vi "testToChangeGainByPSSN.vi"(8 "error in (no error)":errorcluster) -> (0 "error out":errorcluster)   [LabVIEW 2016]
doc: "Test to change the gain value based on the normalized point source sensitivity (PSSN)."
uses:
  ZTAAC/ZTAAC.lvclass
  <vilib>/addons/_JKI Toolkits/Caraya/classes/Test/Test.lvclass
  <vilib>/addons/_JKI Toolkits/Caraya/classes/Assert/Assert.lvclass
panel:
  in  "ZTAAC.lvclass":refnum<class "ZTAAC.lvclass">
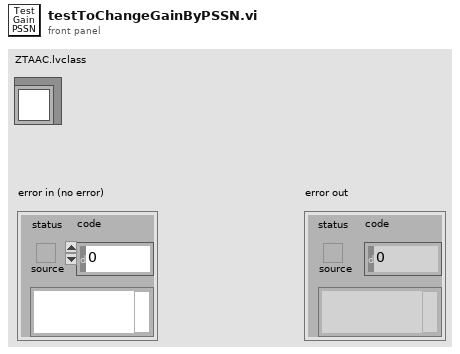
[diagram p1: front panel]
types:
  T1 = typedef "OfcFunc.lvlib/InstName.ctl" = enum16{"lsst", "comcam"}
  T2 = cluster{"Config Dir":path, "Inst Name":T1, "OptStateEsti Config File Name":string, "Mapping File Name":string, "Wavelength Table":string, "Intrinc Zk File Name":string, "y2 Corection File Name":string, "Index DOF File Name":string, "OptCtrl Config File Name":string, "State 0 File Name":string, "Weighting File Name":string, "PSSN Alpha File Name":string, "Authority Files":cluster{"Rigid Body Stroke File":string, "M1M3 Subsystem":cluster{"Mirror":string, "Actuatro Force File":string}, "M2 Subsystem":cluster{"Mirror":string, "Actuatro Force File":string}, "Num of Bending Mode":i32}, "Sensor Id to Name File Name":string, "Truncation Threshold":dbl, "Default Gain":dbl, "FWHM Threshold (arcsec)":dbl}
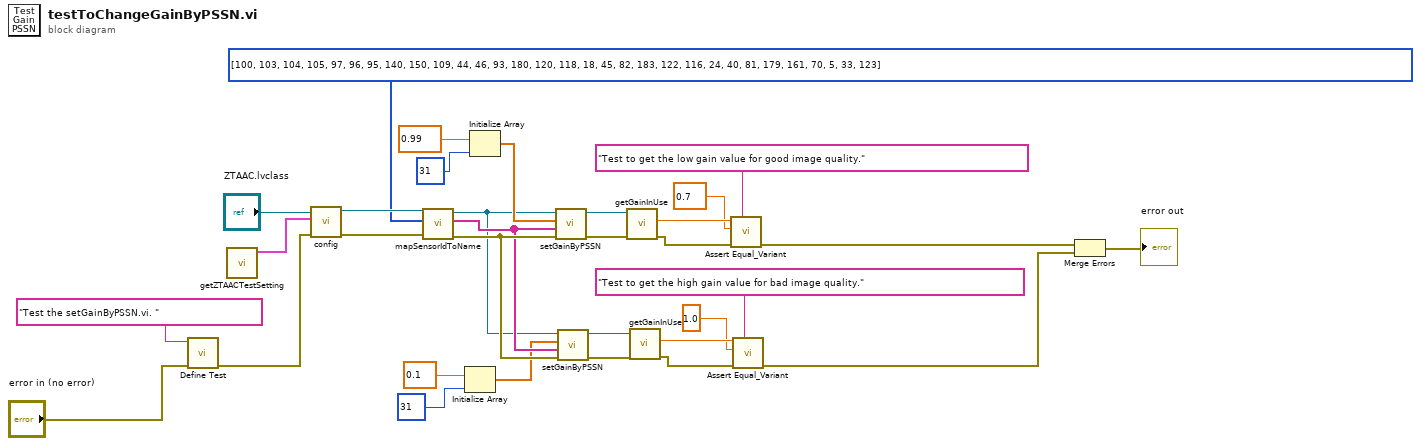
[diagram p0: block diagram]
diagram:
  n1 = call <vilib>:"Define Test.vi"("error in (no error)"="error in (no error)", "Label (VI Title)"="Test the setGainByPSSN.vi. ") -> ("error out"=w13:errorcluster)  [unwired: 9 in]
  n2 = call "getZTAACTestSetting.vi"() -> ("Test Setting"=w1:T2)  [unwired: 11 in]
  n3 = call "config.vi"("error in (no error)"=w13, "ZTAAC Configuration"=w1, "ZTAAC in"="ZTAAC.lvclass") -> ("error out"=w23:errorcluster, "ZTAAC out"=w25:refnum<class "ZTAAC.lvclass">)  [unwired: 7 in]
  n4 = call "mapSensorIdToName.vi"("error in (no error)"=w23, "Sensor Id"=i32[] [100, 103, 104, 105, 97, 96, 95, 140, 150, 109, 44, 46, 93, 180, 120, 118, 18, 45, 82, 183, 122, 116, 24, 40, 81, 179, 161, 70, 5, 33, 123], "ZTAAC in"=w25) -> ("error out"=w21:errorcluster, "Sensor Name"=w20:string[], "ZTAAC out"=w16:refnum<class "ZTAAC.lvclass">)  [unwired: 5 in, 1 out]
  n5 = Initialize Array(0.1 ("element"), 31 ("dimension size")) -> (w19:dbl[])
  n6 = Initialize Array(0.99 ("element"), 31 ("dimension size")) -> (w27:dbl[])
  n7 = call "setGainByPSSN.vi"("error in (no error)"=w21, "Sensor Name"=w20, "PSSN"=w27, "ZTAAC in"=w16) -> ("error out"=w22:errorcluster, "ZTAAC out"=w26:refnum<class "ZTAAC.lvclass">)  [unwired: 6 in]
  n8 = call "setGainByPSSN.vi"("error in (no error)"=w21, "Sensor Name"=w20, "PSSN"=w19, "ZTAAC in"=w16) -> ("error out"=w17:errorcluster, "ZTAAC out"=w18:refnum<class "ZTAAC.lvclass">)  [unwired: 6 in]
  n9 = call "getGainInUse.vi"("error in (no error)"=w22, "ZTAAC in"=w26) -> ("error out"=w10:errorcluster, "Gain in Use"=w12:dbl)  [unwired: 7 in, 1 out]
  n10 = call "getGainInUse.vi"("error in (no error)"=w17, "ZTAAC in"=w18) -> ("error out"=w7:errorcluster, "Gain in Use"=w9:dbl)  [unwired: 7 in, 1 out]
  n11 = call <vilib>:"Assert Equal_Variant.vi"("Label"="Test to get the low gain value for good image quality.", "error in (no error)"=w10, "Y"=0.7 ("element"), "X"=w12) -> ("error out"=w6:errorcluster)  [unwired: 7 in]
  n12 = call <vilib>:"Assert Equal_Variant.vi"("Label"="Test to get the high gain value for bad image quality.", "error in (no error)"=w7, "Y"=1.0 ("element"), "X"=w9) -> ("error out"=w5:errorcluster)  [unwired: 7 in]
  n13 = Merge Errors(w6, w5) -> (→"error out":errorcluster)
